vi "Disable All Outputs.vi"(8 "error in":errorcluster, 11 "36234A in":refnum<class "36234A.lvclass">) -> (0 "error out":errorcluster, 3 "36234A out":refnum<class "36234A.lvclass">)   [LabVIEW 2019, in "36234A.lvlib" / "36234A.lvclass"]
uses:
  Library/36234A.lvclass
  C:/Users/Public/Documents/Development/builds/Instruments/PowerSupply.lvlibp/Library/PowerSupply.lvclass
  builds/Instruments/PowerSupply.lvlibp/Private/Accessors/Read Number of Channels.vi
  builds/Instruments/PowerSupply.lvlibp/Accessors/Write Active Channel.vi
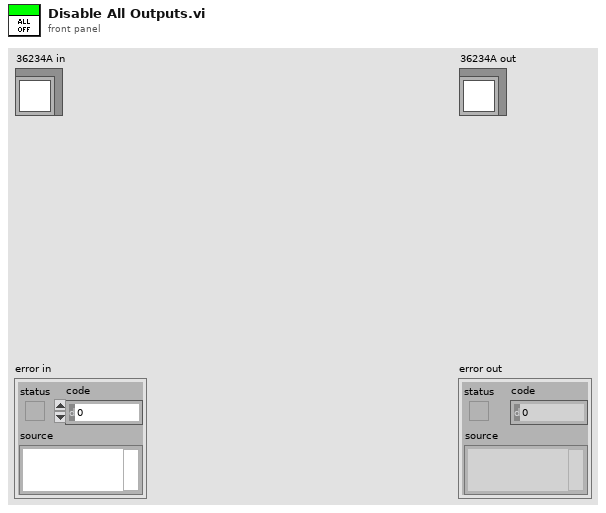
[diagram p1: front panel]
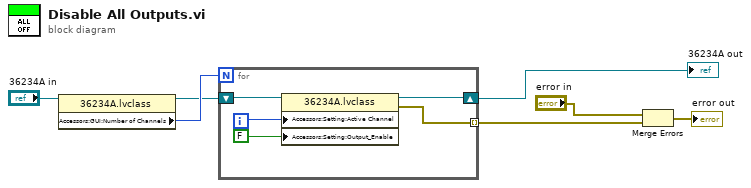
[diagram p0: block diagram]
diagram:
  n1 = property class="36234A.lvclass"(reference="36234A in") -> (reference out=w6:refnum<class "36234A.lvclass">, "Accessors:GUI:Number of Channels"=w7:i32)  [unwired: 1 in, 1 out]
  n2 = for {
    N: w7 -> [_]
    shift-right: [w9] -> w4
    shift-left: w6 -> [w12]
    tunnel: [w8] -> w3 mode=indexing
    i -> [w11]
    n3 = property class="36234A.lvclass"(reference=w12, "Accessors:Setting:Active Channel"=w11, "Accessors:Setting:Output_Enable"=FALSE ("Supply:Settings:Output_Enable")) -> (reference out=w9:refnum<class "36234A.lvclass">, error out=w8:errorcluster)  [unwired: 1 in]
  }
  "36234A out" <- w4
  n4 = Merge Errors("error in", w3) -> (→"error out":errorcluster)
